vi "gh-cli Release View.vi"(8 "error in (no error)":errorcluster, 10 "Options":string, 11 "Git in":refnum<class "Git.lvclass">) -> (0 "error out":errorcluster, 2 "standard output":string, 3 "Git out":refnum<class "Git.lvclass">)   [LabVIEW 2019, in "Git.lvclass"]
doc: "gh release view [<b>Options</b>]: View information about a GitHub Release.\n\n<b>Options</b>\n[<tag>]: Without an explicit tag name argument, the latest release in the project is shown.\n-q, --jq <expression>: Filter JSON output using a jq expression\n--json <fields>: Output JSON with the specified fields\n-t, --template <string>: Format JSON output using a Go template\n-w, --web: Open the release in the browser\n-R, --repo <[HOST/]OWNER/REPO>: Select another repository using the [HOST/]OWNER/REPO format \n\nhttps://cli.github.com/manual"
uses:
  Git.lvclass
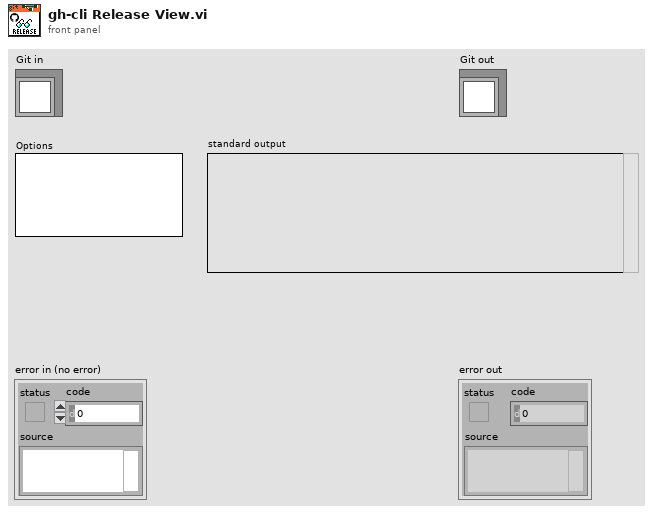
[diagram p1: front panel]
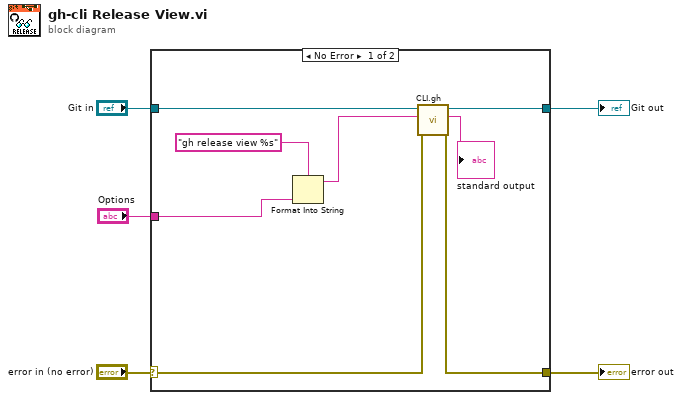
[diagram p0: block diagram]
diagram:
  n1 = case shown="No Error" "error in (no error)" {
    selector: "error in (no error)" -> [w11 w15]
    tunnel: [w10 w15] -> w4
    tunnel: [w12 w14] -> w2
    tunnel: "Git in" -> [w13 w14]
    tunnel: "Options" -> [w7 _]
    frame No Error {
      n2 = Format Into String(format string="gh release view %s", w7) -> (resulting string=w6:string)  [unwired: 2 in, 1 out]
      n3 = call "CLI.gh.vi"("error in (no error)"=w11, "Command"=w6, "Git in"=w13) -> ("error out"=w10:errorcluster, "standard output"=→"standard output":string, "Git out"=w12:refnum<class "Git.lvclass">)  [unwired: 4 in, 2 out]
    }
    frame Error {
    }
  }
  "error out" <- w4
  "Git out" <- w2
